vi "Class - Properties.vi"(7 "Msg Chain":string, 8 "error in (no error)":errorcluster {"code" format="Error %.0f"}, 10 "Classes":refnum<class "Class Documentation.lvclass">[](array[class]), 11 "VIDoc Printer - Confluence In":refnum<class "VIDoc Printer - Confluence.lvclass">) -> (0 "error out":errorcluster {"code" format="Error %.0f"}, 3 "VIDoc Printer - Confluence Out":refnum<class "VIDoc Printer - Confluence.lvclass">)   [LabVIEW 2023, in "VIDoc Printer - Confluence.lvlib" / "VIDoc Printer - Confluence.lvclass"]
uses:
  VIDoc Printer - Confluence.lvclass
  C:/projects/DMC/Tooling/Git-Action-Service/Source/Documentation Generation/Printers/Printer/VIDoc Printer.lvclass
  Parsing/Class Documentation/Class Documentation.lvclass
  Parsing/Class Documentation/Class Documentation.lvclass/Class Documentation.ctl
  Confluence Formatting/Types/Format Combo Box.ctl
  VIDoc Printer - Confluence.lvclass/VIDoc Printer - Confluence.ctl
  Parsing/Class Documentation/Get Parent Classes.vi
  Parsing/Class Documentation/Get Parent Interfaces.vi
  Parsing/Class Documentation/Get Parent Libraries.vi
  Parsing/Class Documentation/Get Class_Library.vi
  Parsing/Class Documentation/Get Name.vi
  Parsing/Class Documentation/Get Total Data Size.vi
  Printer/VIDoc Printer.lvclass
  UI Interaction/UI Interaction.lvclass
  Confluence Formatting/Confluence Formatting.lvlib
  C:/projects/DMC/Tooling/Git-Action-Service/Source/Documentation Generation/Printers/Confluence Printer/VIDoc Printer - Confluence.lvclass
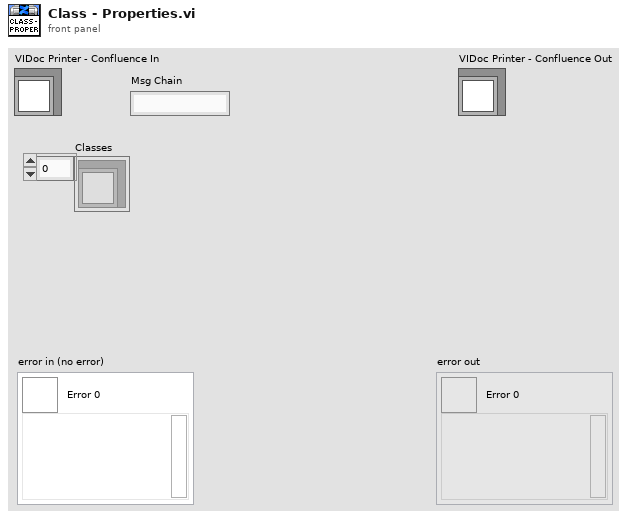
[diagram p1: front panel]
types:
  T1 = typedef "Confluence Formatting.lvlib/Format Combo Box.ctl" = string
  T2 = typedef "VIDoc Parsing.lvlib/Base Class Info Cluster.ctl" = cluster{"Name":string, "Icon":T3, "Version":cluster{"Major":u16, "Minor":u16, "Fix":u16, "Build":u16}, "Description":string, "Friends":string[], "ChildRefsRestricted":bool, "TransferMustOverrides":bool, "Path":path, "Qualified Name":string, "Class Scope":enum32{"invalid scope", "public", "private", "protected", "community"}}
  T3 = typedef "imagedata.ctl" = cluster{"image type":i32, "image depth":i32, "image":u8[], "mask":u8[], "colors":u32[], "Rectangle":cluster{"left":i16, "top":i16, "right":i16, "bottom":i16}}
  T4 = typedef "NI.Parent Library Information.ctl" = cluster{"qualified name":string, "localized name":string, "path":path, "parent library kind":T5}
  T5 = typedef "NI.Parent Library Kind.ctl" = enum32{"unknown", "class", "interface"}
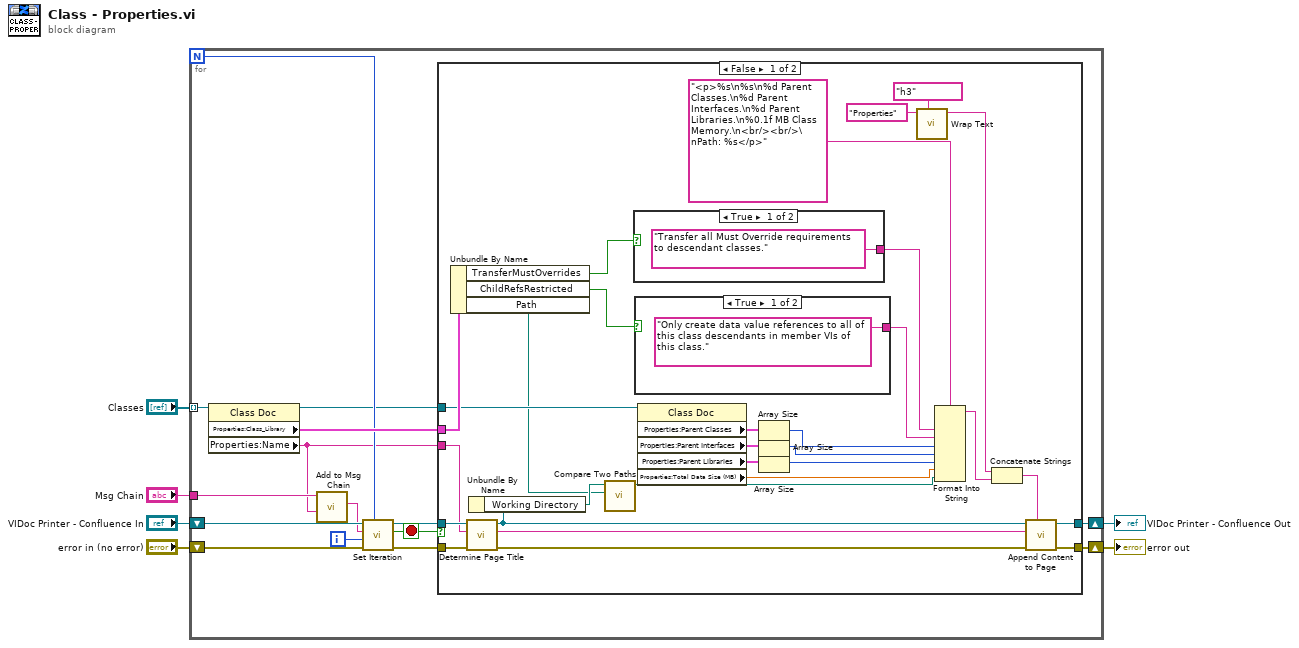
[diagram p0: block diagram]
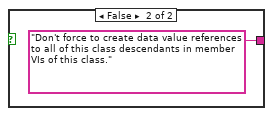
[diagram p2: hidden frame]
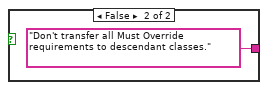
[diagram p3: hidden frame]
diagram:
  n1 = for {
    N -> [w13]
    shift-right: [w19] -> w2
    shift-left: "error in (no error)" -> [w16]
    shift-right: [w20] -> w1
    shift-left: "VIDoc Printer - Confluence In" -> [w17]
    tunnel: "Classes" -> [w21] mode=indexing
    tunnel: "Msg Chain" -> [w11]
    i -> [w12]
    stop <- w8 stop-if-true
    n2 = property class="Class Doc"(reference=w21) -> (reference out=w7:refnum<class "Class Documentation.lvclass">, "Properties:Class_Library"=w18:T2, "Properties:Name"=w10:string)  [unwired: 1 in, 1 out]
    n3 = call "Add to Msg Chain.vi"("New"=w10, "Msg Chain in"=w11) -> ("Msg Chain out"=w9:string)  [unwired: 9 in]
    n4 = call "Set Iteration.vi"("Progress Max"=w13, "error in (no error)"=w16, "Progress Value"=w12, "Message (No Message Update)"=w9, "VIDoc Printer In"=w17) -> ("error out"=w14:errorcluster, "Abort?"=w8:bool, "VIDoc Printer Out"=w15:refnum<class "VIDoc Printer - Confluence.lvclass">)  [unwired: 4 in]
    n5 = case shown="False" w8 {
      tunnel: [w49 w56] -> w20
      tunnel: [w48 w57] -> w19
      tunnel: w18 -> [w28 _]
      tunnel: w15 -> [w44 w56]
      tunnel: w14 -> [w43 w57]
      tunnel: w10 -> [w42 _]
      tunnel: w7 -> [w27 _]
      frame False {
        n6 = Unbundle By Name(w28) -> ("TransferMustOverrides"=w37:bool, "ChildRefsRestricted"=w38:bool, "Path"=w23:path)
        n7 = call "Determine Page Title.vi"("error in (no error)"=w43, "Name"=w42, "VIDoc Printer - Confluence In"=w44) -> ("error out"=w50:errorcluster, "Page Title"=w51:string, "VIDoc Printer - Confluence Out"=w25:refnum<class "VIDoc Printer - Confluence.lvclass">)  [unwired: 5 in, 1 out]
        n8 = Unbundle By Name(w25) -> ("Working Directory"=w24:path)
        n9 = call <vilib>:"Compare Two Paths.vi"("Path 2"=w23, "Path 1"=w24) -> ("Relative Path from 1 to 2"=w22:path)  [unwired: 6 in, 3 out]
        n10 = case shown="True" w37 {
          tunnel: ["Transfer all Must Override requirements to descendant classes." "Don't transfer all Must Override requirements to descendant classes."] -> w39
          frame True {
          }
          frame False {
          }
        }
        n11 = case shown="True" w38 {
          tunnel: ["Only create data value references to all of this class descendants in member VIs of this class." "Don't force to create data value references to all of this class descendants in member VIs of this class."] -> w40
          frame True {
          }
          frame False {
          }
        }
        n12 = property class="Class Doc"(reference=w27) -> ("Properties:Parent Classes"=w30:T2[], "Properties:Parent Interfaces"=w31:T2[], "Properties:Parent Libraries"=w32:T4[], "Properties:Total Data Size (MB)"=w34:dbl)  [unwired: 1 in, 2 out]
        n13 = Array Size(array=w30) -> (size(s)=w36:i32)
        n14 = Array Size(array=w31) -> (size(s)=w35:i32)
        n15 = Array Size(array=w32) -> (size(s)=w33:i32)
        n16 = call "Wrap Text.vi"("Formatting"=T1 "h3", "String"="Properties") -> ("Wrapped String"=w46:string)  [unwired: 8 in, 1 out]
        n17 = Format Into String(format string="<p>%s\n%s\n%d Parent Classes.\n%d Parent Interfaces.\n%d Parent Libraries.\n%0.1f MB Class Memory.\n<br/><br/>\nPath: %s</p>", w39, w40, w36, w35, w33, w34, w22) -> (resulting string=w26:string)  [unwired: 2 in, 1 out]
        n18 = Concatenate Strings(w46, w26) -> (w45:string)
        n19 = call "Append Content to Page.vi"("Page Content"=w45, "error in (no error)"=w50, "Page Title"=w51, "VIDoc Printer - Confluence In"=w25) -> ("error out"=w48:errorcluster, "VIDoc Printer - Confluence Out"=w49:refnum<class "VIDoc Printer - Confluence.lvclass">)  [unwired: 6 in]
      }
      frame True {
      }
    }
  }
  "error out" <- w2
  "VIDoc Printer - Confluence Out" <- w1
